vi "test TCX read (installed 71).vi"() -> ()   [LabVIEW 2011] (continued)
sion/v2\"><Watts>118</Watts></TPX></Extensions></Trackpoint><Trackpoint><Time>2008-03-03T13:49:30Z</Time><Position><LatitudeDegrees>35.887382</LatitudeDegrees><LongitudeDegrees>-78.945030</LongitudeDegrees></Position><AltitudeMeters>85.695</AltitudeMeters><DistanceMeters>793.797</DistanceMeters><Cadence>84</Cadence><Extensions><TPX xmlns=\"http://www.garmin.com/xmlschemas/ActivityExtension/v2\"><Watts>105</Watts></TPX></Extensions></Trackpoint><Trackpoint><Time>2008-03-03T13:49:31Z</Time><Position><LatitudeDegrees>35.887368</LatitudeDegrees><LongitudeDegrees>-78.944943</LongitudeDegrees></Position><AltitudeMeters>85.695</AltitudeMeters><DistanceMeters>801.819</DistanceMeters><Cadence>84</Cadence><Extensions><TPX xmlns=\"http://www.garmin.com/xmlschemas/ActivityExtension/v2\"><Watts>104</Watts></TPX></Extensions></Trackpoint><Trackpoint><Time>2008-03-03T13:49:32Z</Time><Position><LatitudeDegrees>35.887352</LatitudeDegrees><LongitudeDegrees>-78.944857</LongitudeDegrees></Position><AltitudeMeters>85.695</AltitudeMeters><DistanceMeters>809.764</DistanceMeters><Cadence>81</Cadence><Extensions><TPX xmlns=\"http://www.garmin.com/xmlschemas/ActivityExtension/v2\"><Watts>123</Watts></TPX></Extensions></Trackpoint><Trackpoint><Time>2008-03-03T13:49:33Z</Time><Position><LatitudeDegrees>35.887335</LatitudeDegrees><LongitudeDegrees>-78.944773</LongitudeDegrees></Position><AltitudeMeters>85.695</AltitudeMeters><DistanceMeters>817.588</DistanceMeters><Cadence>81</Cadence><Extensions><TPX xmlns=\"http://www.garmin.com/xmlschemas/ActivityExtension/v2\"><Watts>122</Watts></TPX></Extensions></Trackpoint><Trackpoint><Time>2008-03-03T13:49:34Z</Time><Position><LatitudeDegrees>35.887319</LatitudeDegrees><LongitudeDegrees>-78.944691</LongitudeDegrees></Position><AltitudeMeters>86.175</AltitudeMeters><DistanceMeters>825.167</DistanceMeters><Cadence>76</Cadence><Extensions><TPX xmlns=\"http://www.garmin.com/xmlschemas/ActivityExtension/v2\"><Watts>160</Watts></TPX></Extensions></Trackpoint><Trackpoint><Time>2008-03-03T13:49:35Z</Time><Position><LatitudeDegrees>35.887303</LatitudeDegrees><LongitudeDegrees>-78.944612</LongitudeDegrees></Position><AltitudeMeters>86.656</AltitudeMeters><DistanceMeters>832.484</DistanceMeters><Cadence>74</Cadence><Extensions><TPX xmlns=\"http://www.garmin.com/xmlschemas/ActivityExtension/v2\"><Watts>198</Watts></TPX></Extensions></Trackpoint><Trackpoint><Time>2008-03-03T13:49:36Z</Time><Position><LatitudeDegrees>35.887288</LatitudeDegrees><LongitudeDegrees>-78.944536</LongitudeDegrees></Position><AltitudeMeters>86.656</AltitudeMeters><DistanceMeters>839.529</DistanceMeters><Cadence>74</Cadence><Extensions><TPX xmlns=\"http://www.garmin.com/xmlschemas/ActivityExtension/v2\"><Watts>196</Watts></TPX></Extensions></Trackpoint><Trackpoint><Time>2008-03-03T13:49:37Z</Time><Position><LatitudeDegrees>35.887275</LatitudeDegrees><LongitudeDegrees>-78.944463</LongitudeDegrees></Position><AltitudeMeters>87.137</AltitudeMeters><DistanceMeters>846.312</DistanceMeters><Cadence>70</Cadence><Extensions><TPX xmlns=\"http://www.garmin.com/xmlschemas/ActivityExtension/v2\"><Watts>222</Watts></TPX></Extensions></Trackpoint><Trackpoint><Time>2008-03-03T13:49:38Z</Time><Position><LatitudeDegrees>35.887261</LatitudeDegrees><LongitudeDegrees>-78.944394</LongitudeDegrees></Position><AltitudeMeters>87.137</AltitudeMeters><DistanceMeters>852.718</DistanceMeters><Cadence>66</Cadence><Extensions><TPX xmlns=\"http://www.garmin.com/xmlschemas/ActivityExtension/v2\"><Watts>181</Watts></TPX></Extensions></Trackpoint><Trackpoint><Time>2008-03-03T13:49:39Z</Time><Position><LatitudeDegrees>35.887248</LatitudeDegrees><LongitudeDegrees>-78.944330</LongitudeDegrees></Position><AltitudeMeters>87.137</AltitudeMeters><DistanceMeters>858.649</DistanceMeters><Cadence>66</Cadence><Extensions><TPX xmlns=\"http://www.garmin.com/xmlschemas/ActivityExtension/v2\"><Watts>181</Watts></TPX></Extensions></Trackpoint><Trackpoint><Time>2008-03-03T13:49:40Z</Time><Position><LatitudeDegrees>35.887233</LatitudeDegrees><LongitudeDegrees>-78.944273</LongitudeDegrees></Position><AltitudeMeters>87.137</AltitudeMeters><DistanceMeters>863.967</DistanceMeters><Cadence>26</Cadence><Extensions><TPX xmlns=\"http://www.garmin.com/xmlschemas/ActivityExtension/v2\"><Watts>4</Watts></TPX></Extensions></Trackpoint><Trackpoint><Time>2008-03-03T13:49:41Z</Time><Position><LatitudeDegrees>35.887206</LatitudeDegrees><LongitudeDegrees>-78.944231</LongitudeDegrees></Position><AltitudeMeters>87.617</AltitudeMeters><DistanceMeters>868.672</DistanceMeters><Cadence>53</Cadence><Extensions><TPX xmlns=\"http://www.garmin.com/xmlschemas/ActivityExtension/v2\"><Watts>162</Watts></TPX></Extensions></Trackpoint><Trackpoint><Time>2008-03-03T13:49:42Z</Time><Position><LatitudeDegrees>35.887168</LatitudeDegrees><LongitudeDegrees>-78.944206</LongitudeDegrees></Position><AltitudeMeters>88.098</AltitudeMeters><DistanceMeters>873.489</DistanceMeters><Cadence>53</Cadence><Extensions><TPX xmlns=\"http://www.garmin.com/xmlschemas/ActivityExtension/v2\"><Watts>215</Watts></TPX></Extensions></Trackpoint><Trackpoint><Time>2008-03-03T13:49:43Z</Time><Position><LatitudeDegrees>35.887123</LatitudeDegrees><LongitudeDegrees>-78.944197</LongitudeDegrees></Position><AltitudeMeters>88.098</AltitudeMeters><DistanceMeters>878.466</DistanceMeters><Cadence>53</Cadence><Extensions><TPX xmlns=\"http://www.garmin.com/xmlschemas/ActivityExtension/v2\"><Watts>227</Watts></TPX></Extensions></Trackpoint><Trackpoint><Time>2008-03-03T13:49:44Z</Time><Position><LatitudeDegrees>35.887076</LatitudeDegrees><LongitudeDegrees>-78.944202</LongitudeDegrees></Position><AltitudeMeters>88.579</AltitudeMeters><DistanceMeters>883.720</DistanceMeters><Cadence>54</Cadence><Extensions><TPX xmlns=\"http://www.garmin.com/xmlschemas/ActivityExtension/v2\"><Watts>313</Watts></TPX></Extensions></Trackpoint><Trackpoint><Time>2008-03-03T13:49:45Z</Time><Position><LatitudeDegrees>35.887028</LatitudeDegrees><LongitudeDegrees>-78.944215</LongitudeDegrees></Position><AltitudeMeters>88.579</AltitudeMeters><DistanceMeters>889.221</DistanceMeters><Cadence>55</Cadence><Extensions><TPX xmlns=\"http://www.garmin.com/xmlschemas/ActivityExtension/v2\"><Watts>319</Watts></TPX></Extensions></Trackpoint><Trackpoint><Time>2008-03-03T13:49:46Z</Time><Position><LatitudeDegrees>35.886978</LatitudeDegrees><LongitudeDegrees>-78.944234</LongitudeDegrees></Position><AltitudeMeters>88.579</AltitudeMeters><DistanceMeters>895.079</DistanceMeters><Cadence>59</Cadence><Extensions><TPX xmlns=\"http://www.garmin.com/xmlschemas/ActivityExtension/v2\"><Watts>307</Watts></TPX></Extensions></Trackpoint><Trackpoint><Time>2008-03-03T13:49:47Z</Time><Position><LatitudeDegrees>35.886925</LatitudeDegrees><LongitudeDegrees>-78.944254</LongitudeDegrees></Position><AltitudeMeters>89.059</AltitudeMeters><DistanceMeters>901.230</DistanceMeters><Cadence>64</Cadence><Extensions><TPX xmlns=\"http://www.garmin.com/xmlschemas/ActivityExtension/v2\"><Watts>315</Watts></TPX></Extensions></Trackpoint><Trackpoint><Time>2008-03-03T13:49:48Z</Time><Position><LatitudeDegrees>35.886870</LatitudeDegrees><LongitudeDegrees>-78.944274</LongitudeDegrees></Position><AltitudeMeters>89.059</AltitudeMeters><DistanceMeters>907.640</DistanceMeters><Cadence>64</Cadence><Extensions><TPX xmlns=\"http://www.garmin.com/xmlschemas/ActivityExtension/v2\"><Watts>314</Watts></TPX></Extensions></Trackpoint><Trackpoint><Time>2008-03-03T13:49:49Z</Time><Position><LatitudeDegrees>35.886813</LatitudeDegrees><LongitudeDegrees>-78.944295</LongitudeDegrees></Position><AltitudeMeters>89.059</AltitudeMeters><DistanceMeters>914.208</DistanceMeters><Cadence>67</Cadence><Extensions><TPX xmlns=\"http://www.garmin.com/xmlschemas/ActivityExtension/v2\"><Watts>312</Watts></TPX></Extensions></Trackpoint><Trackpoint><Time>2008-03-03T13:49:50Z</Time><Position><LatitudeDegrees>35.886755</LatitudeDegrees><LongitudeDegrees>-78.944316</LongitudeDegrees></Position><AltitudeMeters>89.540</AltitudeMeters><DistanceMeters>920.951</DistanceMeters><Cadence>69</Cadence><Extensions><TPX xmlns=\"http://www.garmin.com/xmlschemas/ActivityExtension/v2\"><Watts>307</Watts></TPX></Extensions></Trackpoint><Trackpoint><Time>2008-03-03T13:49:51Z</Time><Position><LatitudeDegrees>35.886696</LatitudeDegrees><LongitudeDegrees>-78.944339</LongitudeDegrees></Position><AltitudeMeters>89.540</AltitudeMeters><DistanceMeters>927.813</DistanceMeters><Cadence>70</Cadence><Extensions><TPX xmlns=\"http://www.garmin.com/xmlschemas/ActivityExtension/v2\"><Watts>284</Watts></TPX></Extensions></Trackpoint><Trackpoint><Time>2008-03-03T13:49:52Z</Time><Position><LatitudeDegrees>35.886636</LatitudeDegrees><LongitudeDegrees>-78.944362</LongitudeDegrees></Position><AltitudeMeters>90.021</AltitudeMeters><DistanceMeters>934.772</DistanceMeters><Cadence>71</Cadence><Extensions><TPX xmlns=\"http://www.garmin.com/xmlschemas/ActivityExtension/v2\"><Watts>269</Watts></TPX></Extensions></Trackpoint><Trackpoint><Time>2008-03-03T13:49:53Z</Time><Position><LatitudeDegrees>35.886575</LatitudeDegrees><LongitudeDegrees>-78.944386</LongitudeDegrees></Position><AltitudeMeters>90.021</AltitudeMeters><DistanceMeters>941.893</DistanceMeters><Cadence>72</Cadence><Extensions><TPX xmlns=\"http://www.garmin.com/xmlschemas/ActivityExtension/v2\"><Watts>267</Watts></TPX></Extensions></Trackpoint><Trackpoint><Time>2008-03-03T13:49:54Z</Time><Position><LatitudeDegrees>35.886513</LatitudeDegrees><LongitudeDegrees>-78.944411</LongitudeDegrees></Position><AltitudeMeters>90.021</AltitudeMeters><DistanceMeters>949.165</DistanceMeters><Cadence>73</Cadence><Extensions><TPX xmlns=\"http://www.garmin.com/xmlschemas/ActivityExtension/v2\"><Watts>268</Watts></TPX></Extensions></Trackpoint><Trackpoint><Time>2008-03-03T13:49:55Z</Time><Position><LatitudeDegrees>35.886450</LatitudeDegrees><LongitudeDegrees>-78.944438</LongitudeDegrees></Position><AltitudeMeters>90.501</AltitudeMeters><DistanceMeters>956.557</DistanceMeters><Cadence>74</Cadence><Extensions><TPX xmlns=\"http://www.garmin.com/xmlschemas/ActivityExtension/v2\"><Watts>281</Watts></TPX></Extensions></Trackpoint><Trackpoint><Time>2008-03-03T13:49:56Z</Time><Position><LatitudeDegrees>35.886386</LatitudeDegrees><LongitudeDegrees>-78.944466</LongitudeDegrees></Position><AltitudeMeters>90.501</AltitudeMeters><DistanceMeters>964.022</DistanceMeters><Cadence>75</Cadence><Extensions><TPX xmlns=\"http://www.garmin.com/xmlschemas/ActivityExtension/v2\"><Watts>280</Watts></TPX></Extensions></Trackpoint><Trackpoint><Time>2008-03-03T13:49:57Z</Time><Position><LatitudeDegrees>35.886323</LatitudeDegrees><LongitudeDegrees>-78.944495</LongitudeDegrees></Position><AltitudeMeters>90.501</AltitudeMeters><DistanceMeters>971.556</DistanceMeters><Cadence>76</Cadence><Extensions><TPX xmlns=\"http://www.garmin.com/xmlschemas/ActivityExtension/v2\"><Watts>255</Watts></TPX></Extensions></Trackpoint><Trackpoint><Time>2008-03-03T13:49:58Z</Time><Position><LatitudeDegrees>35.886260</LatitudeDegrees><LongitudeDegrees>-78.944528</LongitudeDegrees></Position><AltitudeMeters>90.501</AltitudeMeters><DistanceMeters>979.102</DistanceMeters><Cadence>76</Cadence><Extensions><TPX xmlns=\"http://www.garmin.com/xmlschemas/ActivityExtension/v2\"><Watts>221</Watts></TPX></Extensions></Trackpoint><Trackpoint><Time>2008-03-03T13:49:59Z</Time><Position><LatitudeDegrees>35.886198</LatitudeDegrees><LongitudeDegrees>-78.944565</LongitudeDegrees></Position><AltitudeMeters>90.501</AltitudeMeters><DistanceMeters>986.796</DistanceMeters><Cadence>78</Cadence><Extensions><TPX xmlns=\"http://www.garmin.com/xmlschemas/ActivityExtension/v2\"><Watts>223</Watts></TPX></Extensions></Trackpoint><Trackpoint><Time>2008-03-03T13:50:00Z</Time><Position><LatitudeDegrees>35.886135</LatitudeDegrees><LongitudeDegrees>-78.944606</LongitudeDegrees></Position><AltitudeMeters>90.501</AltitudeMeters><DistanceMeters>994.741</DistanceMeters><Cadence>80</Cadence><Extensions><TPX xmlns=\"http://www.garmin.com/xmlschemas/ActivityExtension/v2\"><Watts>218</Watts></TPX></Extensions></Trackpoint><Trackpoint><Time>2008-03-03T13:50:01Z</Time><Position><LatitudeDegrees>35.886071</LatitudeDegrees><LongitudeDegrees>-78.944649</LongitudeDegrees></Position><AltitudeMeters>90.501</AltitudeMeters><DistanceMeters>1002.808</DistanceMeters><Cadence>81</Cadence><Extensions><TPX xmlns=\"http://www.garmin.com/xmlschemas/ActivityExtension/v2\"><Watts>218</Watts></TPX></Extensions></Trackpoint><Trackpoint><Time>2008-03-03T13:50:02Z</Time><Position><LatitudeDegrees>35.886008</LatitudeDegrees><LongitudeDegrees>-78.944696</LongitudeDegrees></Position><AltitudeMeters>90.501</AltitudeMeters><DistanceMeters>1011.004</DistanceMeters><Cadence>77</Cadence><Extensions><TPX xmlns=\"http://www.garmin.com/xmlschemas/ActivityExtension/v2\"><Watts>191</Watts></TPX></Extensions></Trackpoint><Trackpoint><Time>2008-03-03T13:50:03Z</Time><Position><LatitudeDegrees>35.885946</LatitudeDegrees><LongitudeDegrees>-78.944747</LongitudeDegrees></Position><AltitudeMeters>90.501</AltitudeMeters><DistanceMeters>1019.345</DistanceMeters><Cadence>77</Cadence><Extensions><TPX xmlns=\"http://www.garmin.com/xmlschemas/ActivityExtension/v2\"><Watts>191</Watts></TPX></Extensions></Trackpoint><Trackpoint><Time>2008-03-03T13:50:04Z</Time><Position><LatitudeDegrees>35.885883</LatitudeDegrees><LongitudeDegrees>-78.944801</LongitudeDegrees></Position><AltitudeMeters>90.021</AltitudeMeters><DistanceMeters>1027.811</DistanceMeters><Cadence>77</Cadence><Extensions><TPX xmlns=\"http://www.garmin.com/xmlschemas/ActivityExtension/v2\"><Watts>162</Watts></TPX></Extensions></Trackpoint><Trackpoint><Time>2008-03-03T13:50:05Z</Time><Position><LatitudeDegrees>35.885821</LatitudeDegrees><LongitudeDegrees>-78.944859</LongitudeDegrees></Position><AltitudeMeters>90.021</AltitudeMeters><DistanceMeters>1036.483</DistanceMeters><Cadence>77</Cadence><Extensions><TPX xmlns=\"http://www.garmin.com/xmlschemas/ActivityExtension/v2\"><Watts>163</Watts></TPX></Extensions></Trackpoint><Trackpoint><Time>2008-03-03T13:50:06Z</Time><Position><LatitudeDegrees>35.885758</LatitudeDegrees><LongitudeDegrees>-78.944919</LongitudeDegrees></Position><AltitudeMeters>90.021</AltitudeMeters><DistanceMeters>1045.314</DistanceMeters><Cadence>79</Cadence><Extensions><TPX xmlns=\"http://www.garmin.com/xmlschemas/ActivityExtension/v2\"><Watts>162</Watts></TPX></Extensions></Trackpoint><Trackpoint><Time>2008-03-03T13:50:07Z</Time><Position><LatitudeDegrees>35.885695</LatitudeDegrees><LongitudeDegrees>-78.944981</LongitudeDegrees></Position><AltitudeMeters>90.021</AltitudeMeters><DistanceMeters>1054.269</DistanceMeters><Cadence>80</Cadence><Extensions><TPX xmlns=\"http://www.garmin.com/xmlschemas/ActivityExtension/v2\"><Watts>162</Watts></TPX></Extensions></Trackpoint><Trackpoint><Time>2008-03-03T13:50:08Z</Time><Position><LatitudeDegrees>35.885631</LatitudeDegrees><LongitudeDegrees>-78.945045</LongitudeDegrees></Position><AltitudeMeters>90.021</AltitudeMeters><DistanceMeters>1063.442</DistanceMeters><Cadence>82</Cadence><Extensions><TPX xmlns=\"http://www.garmin.com/xmlschemas/ActivityExtension/v2\"><Watts>160</Watts></TPX></Extensions></Trackpoint><Trackpoint><Time>2008-03-03T13:50:09Z</Time><Position><LatitudeDegrees>35.885567</LatitudeDegrees><LongitudeDegrees>-78.945111</LongitudeDegrees></Position><AltitudeMeters>89.540</AltitudeMeters><DistanceMeters>1072.743</DistanceMeters><Cadence>84</Cadence><Extensions><TPX xmlns=\"http://www.garmin.com/xmlschemas/ActivityExtension/v2\"><Watts>146</Watts></TPX></Extensions></Trackpoint><Trackpoint><Time>2008-03-03T13:50:10Z</Time><Position><LatitudeDegrees>35.885502</LatitudeDegrees><LongitudeDegrees>-78.945178</LongitudeDegrees></Position><AltitudeMeters>90.021</AltitudeMeters><DistanceMeters>1082.148</DistanceMeters><Cadence>84</Cadence><Extensions><TPX xmlns=\"http://www.garmin.com/xmlschemas/ActivityExtension/v2\"><Watts>146</Watts></TPX></Extensions></Trackpoint><Trackpoint><Time>2008-03-03T13:50:11Z</Time><Position><LatitudeDegrees>35.885437</LatitudeDegrees><LongitudeDegrees>-78.945246</LongitudeDegrees></Position><AltitudeMeters>89.540</AltitudeMeters><DistanceMeters>1091.624</DistanceMeters><Cadence>85</Cadence><Extensions><TPX xmlns=\"http://www.garmin.com/xmlschemas/ActivityExtension/v2\"><Watts>138</Watts></TPX></Extensions></Trackpoint><Trackpoint><Time>2008-03-03T13:50:12Z</Time><Position><LatitudeDegrees>35.885372</LatitudeDegrees><LongitudeDegrees>-78.945314</LongitudeDegrees></Position><AltitudeMeters>89.059</AltitudeMeters><DistanceMeters>1101.113</DistanceMeters><Cadence>86</Cadence><Extensions><TPX xmlns=\"http://www.garmin.com/xmlschemas/ActivityExtension/v2\"><Watts>124</Watts></TPX></Extensions></Trackpoint><Trackpoint><Time>2008-03-03T13:50:13Z</Time><Position><LatitudeDegrees>35.885306</LatitudeDegrees><LongitudeDegrees>-78.945381</LongitudeDegrees></Position><AltitudeMeters>89.059</AltitudeMeters><DistanceMeters>1110.635</DistanceMeters><Cadence>86</Cadence><Extensions><TPX xmlns=\"http://www.garmin.com/xmlschemas/ActivityExtension/v2\"><Watts>126</Watts></TPX></Extensions></Trackpoint><Trackpoint><Time>2008-03-03T13:50:14Z</Time><Position><LatitudeDegrees>35.885239</LatitudeDegrees><LongitudeDegrees>-78.945447</LongitudeDegrees></Position><AltitudeMeters>88.579</AltitudeMeters><DistanceMeters>1120.112</DistanceMeters><Cadence>86</Cadence><Extensions><TPX xmlns=\"http://www.garmin.com/xmlschemas/ActivityExtension/v2\"><Watts>124</Watts></TPX></Extensions></Trackpoint><Trackpoint><Time>2008-03-03T13:50:15Z</Time><Position><LatitudeDegrees>35.885174</LatitudeDegrees><LongitudeDegrees>-78.945514</LongitudeDegrees></Position><AltitudeMeters>88.579</AltitudeMeters><DistanceMeters>1129.584</DistanceMeters><Cadence>86</Cadence><Extensions><TPX xmlns=\"http://www.garmin.com/xmlschemas/ActivityExtension/v2\"><Watts>124</Watts></TPX></Extensions></Trackpoint><Trackpoint><Time>2008-03-03T13:50:16Z</Time><Position><LatitudeDegrees>35.885109</LatitudeDegrees><LongitudeDegrees>-78.945582</LongitudeDegrees></Position><AltitudeMeters>89.059</AltitudeMeters><DistanceMeters>1139.016</DistanceMeters><Cadence>86</Cadence><Extensions><TPX xmlns=\"http://www.garmin.com/xmlschemas/ActivityExtension/v2\"><Watts>130</Watts></TPX></Extensions></Trackpoint><Trackpoint><Time>2008-03-03T13:50:17Z</Time><Position><LatitudeDegrees>35.885046</LatitudeDegrees><LongitudeDegrees>-78.945649</LongitudeDegrees></Position><AltitudeMeters>90.021</AltitudeMeters><DistanceMeters>1148.277</DistanceMeters><Cadence>85</Cadence><Extensions><TPX xmlns=\"http://www.garmin.com/xmlschemas/ActivityExtension/v2\"><Watts>131</Watts></TPX></Extensions></Trackpoint><Trackpoint><Time>2008-03-03T13:50:18Z</Time><Position><LatitudeDegrees>35.884985</LatitudeDegrees><LongitudeDegrees>-78.945716</LongitudeDegrees></Position><AltitudeMeters>90.982</AltitudeMeters><DistanceMeters>1157.323</DistanceMeters><Cadence>84</Cadence><Extensions><TPX xmlns=\"http://www.garmin.com/xmlschemas/ActivityExtension/v2\"><Watts>135</Watts></TPX></Extensions></Trackpoint><Trackpoint><Time>2008-03-03T13:50:19Z</Time><Position><LatitudeDegrees>35.884925</LatitudeDegrees><LongitudeDegrees>-78.945781</LongitudeDegrees></Position><AltitudeMeters>89.540</AltitudeMeters><DistanceMeters>1166.191</DistanceMeters><Cadence>81</Cadence><Extensions><TPX xmlns=\"http://www.garmin.com/xmlschemas/ActivityExtension/v2\"><Watts>152</Watts></TPX></Extensions></Trackpoint><Trackpoint><Time>2008-03-03T13:50:20Z</Time><Position><LatitudeDegrees>35.884864</LatitudeDegrees><LongitudeDegrees>-78.945844</LongitudeDegrees></Position><AltitudeMeters>90.501</AltitudeMeters><DistanceMeters>1174.987</DistanceMeters><Cadence>81</Cadence><Extensions><TPX xmlns=\"http://www.garmin.com/xmlschemas/ActivityExtension/v2\"><Watts>151</Watts></TPX></Extensions></Trackpoint><Trackpoint><Time>2008-03-03T13:50:21Z</Time><Position><LatitudeDegrees>35.884808</LatitudeDegrees><LongitudeDegrees>-78.945907</LongitudeDegrees></Position><AltitudeMeters>90.021</AltitudeMeters><DistanceMeters>1183.414</DistanceMeters><Cadence>80</Cadence><Extensions><TPX xmlns=\"http://www.garmin.com/xmlschemas/ActivityExtension/v2\"><Watts>178</Watts></TPX></Extensions></Trackpoint><Trackpoint><Time>2008-03-03T13:50:22Z</Time><Position><LatitudeDegrees>35.884755</LatitudeDegrees><LongitudeDegrees>-78.945968</LongitudeDegrees></Position><AltitudeMeters>89.540</AltitudeMeters><DistanceMeters>1191.446</DistanceMeters><Cadence>79</Cadence><Extensions><TPX xmlns=\"http://www.garmin.com/xmlschemas/ActivityExtension/v2\"><Watts>217</Watts></TPX></Extensions></Trackpoint><Trackpoint><Time>2008-03-03T13:50:23Z</Time><Position><LatitudeDegrees>35.884706</LatitudeDegrees><LongitudeDegrees>-78.946030</LongitudeDegrees></Position><AltitudeMeters>90.021</AltitudeMeters><DistanceMeters>1199.238</DistanceMeters><Cadence>78</Cadence><Extensions><TPX xmlns=\"http://www.garmin.com/xmlschemas/ActivityExtension/v2\"><Watts>287</Watts></TPX></Extensions></Trackpoint><Trackpoint><Time>2008-03-03T13:50:24Z</Time><Position><LatitudeDegrees>35.884650</LatitudeDegrees><LongitudeDegrees>-78.946090</LongitudeDegrees></Position><AltitudeMeters>89.540</AltitudeMeters><DistanceMeters>1207.446</DistanceMeters><Cadence>77</Cadence><Extensions><TPX xmlns=\"http://www.garmin.com/xmlschemas/ActivityExtension/v2\"><Watts>289</Watts></TPX></Extensions></Trackpoint><Trackpoint><Time>2008-03-03T13:50:25Z</Time><Position><LatitudeDegrees>35.884592</LatitudeDegrees><LongitudeDegrees>-78.946148</LongitudeDegrees></Position><AltitudeMeters>90.021</AltitudeMeters><DistanceMeters>1215.693</DistanceMeters><Cadence>75</Cadence><Extensions><TPX xmlns=\"http://www.garmin.com/xmlschemas/ActivityExtension/v2\"><Watts>287</Watts></TPX></Extensions></Trackpoint><Trackpoint><Time>2008-03-03T13:50:26Z</Time><Position><LatitudeDegrees>35.884536</LatitudeDegrees><LongitudeDegrees>-78.946205</LongitudeDegrees></Position><AltitudeMeters>90.021</AltitudeMeters><DistanceMeters>1223.751</DistanceMeters><Cadence>73</Cadence><Extensions><TPX xmlns=\"http://www.garmin.com/xmlschemas/ActivityExtension/v2\"><Watts>295</Watts></TPX></Extensions></Trackpoint><Trackpoint><Time>2008-03-03T13:50:27Z</Time><Position><LatitudeDegrees>35.884483</LatitudeDegrees><LongitudeDegrees>-78.946259</LongitudeDegrees></Position><AltitudeMeters>90.021</AltitudeMeters><DistanceMeters>1231.388</DistanceMeters><Cadence>73</Cadence><Extensions><TPX xmlns=\"http://www.garmin.com/xmlschemas/ActivityExtension/v2\"><Watts>296</Watts></TPX></Extensions></Trackpoint><Trackpoint><Time>2008-03-03T13:50:28Z</Time><Position><LatitudeDegrees>35.884431</LatitudeDegrees><LongitudeDegrees>-78.946311</LongitudeDegrees></Position><AltitudeMeters>90.501</AltitudeMeters><DistanceMeters>1238.840</DistanceMeters><Cadence>71</Cadence><Extensions><TPX xmlns=\"http://www.garmin.com/xmlschemas/ActivityExtension/v2\"><Watts>301</Watts></TPX></Extensions></Trackpoint><Trackpoint><Time>2008-03-03T13:50:29Z</Time><Position><LatitudeDegrees>35.884379</LatitudeDegrees><LongitudeDegrees>-78.946362</LongitudeDegrees></Position><AltitudeMeters>90.501</AltitudeMeters><DistanceMeters>1246.250</DistanceMeters><Cadence>69</Cadence><Extensions><TPX xmlns=\"http://www.garmin.com/xmlschemas/ActivityExtension/v2\"><Watts>306</Watts></TPX></Extensions></Trackpoint><Trackpoint><Time>2008-03-03T13:50:30Z</Time><Position><LatitudeDegrees>35.884325</LatitudeDegrees><LongitudeDegrees>-78.946412</LongitudeDegrees></Position><AltitudeMeters>90.501</AltitudeMeters><DistanceMeters>1253.653</DistanceMeters><Cadence>69</Cadence><Extensions><TPX xmlns=\"http://www.garmin.com/xmlschemas/ActivityExtension/v2\"><Watts>304</Watts></TPX></Extensions></Trackpoint><Trackpoint><Time>2008-03-03T13:50:31Z</Time><Position><LatitudeDegrees>35.884272</LatitudeDegrees><LongitudeDegrees>-78.946462</LongitudeDegrees></Position><AltitudeMeters>90.501</AltitudeMeters><DistanceMeters>1261.132</DistanceMeters><Cadence>68</Cadence><Extensions><TPX xmlns=\"http://www.garmin.com/xmlschemas/ActivityExtension/v2\"><Watts>304</Watts></TPX></Extensions></Trackpoint><Trackpoint><Time>2008-03-03T13:50:32Z</Time><Position><LatitudeDegrees>35.884218</LatitudeDegrees><LongitudeDegrees>-78.946508</LongitudeDegrees></Position><AltitudeMeters>90.501</AltitudeMeters><DistanceMeters>1268.362</DistanceMeters><Cadence>68</Cadence><Extensions><TPX xmlns=\"http://www.garmin.com/xmlschemas/ActivityExtension/v2\"><Watts>300</Watts></TPX></Extensions></Trackpoint><Trackpoint><Time>2008-03-03T13:50:33Z</Time><Position><LatitudeDegrees>35.884164</LatitudeDegrees><LongitudeDegrees>-78.946555</LongitudeDegrees></Position><AltitudeMeters>90.982</AltitudeMeters><DistanceMeters>1275.758</DistanceMeters><Cadence>69</Cadence><Extensions><TPX xmlns=\"http://www.garmin.com/xmlschemas/ActivityExtension/v2\"><Watts>268</Watts></TPX></Extensions></Trackpoint><Trackpoint><Time>2008-03-03T13:50:34Z</Time><Position><LatitudeDegrees>35.884108</LatitudeDegrees><LongitudeDegrees>-78.946601</LongitudeDegrees></Position><AltitudeMeters>91.463</AltitudeMeters><DistanceMeters>1283.255</DistanceMeters><Cadence>69</Cadence><Extensions><TPX xmlns=\"http://www.garmin.com/xmlschemas/ActivityExtension/v2\"><Watts>267</Watts></TPX></Extensions></Trackpoint><Trackpoint><Time>2008-03-03T13:50:35Z</Time><Position><LatitudeDegrees>35.884049</LatitudeDegrees><LongitudeDegrees>-78.946643</LongitudeDegrees></Position><AltitudeMeters>91.463</AltitudeMeters><DistanceMeters>1290.863</DistanceMeters><Cadence>70</Cadence><Extensions><TPX xmlns=\"http://www.garmin.com/xmlschemas/ActivityExtension/v2\"><Watts>248</Watts></TPX></Extensions></Trackpoint><Trackpoint><Time>2008-03-03T13:50:36Z</Time><Position><LatitudeDegrees>35.883988</LatitudeDegrees><LongitudeDegrees>-78.946685</LongitudeDegrees></Position><AltitudeMeters>90.982</AltitudeMeters><DistanceMeters>1298.547</DistanceMeters><Cadence>70</Cadence><Extensions><TPX xmlns=\"http://www.garmin.com/xmlschemas/ActivityExtension/v2\"><Watts>211</Watts></TPX></Extensions></Trackpoint><Trackpoint><Time>2008-03-03T13:50:37Z</Time><Position><LatitudeDegrees>35.883926</LatitudeDegrees><LongitudeDegrees>-78.946726</LongitudeDegrees></Position><AltitudeMeters>90.982</AltitudeMeters><DistanceMeters>1306.398</DistanceMeters><Cadence>71</Cadence><Extensions><TPX xmlns=\"http://www.garmin.com/xmlschemas/ActivityExtension/v2\"><Watts>186</Watts></TPX></Extensions></Trackpoint><Trackpoint><Time>2008-03-03T13:50:38Z</Time><Position><LatitudeDegrees>35.883861</LatitudeDegrees><LongitudeDegrees>-78.946762</LongitudeDegrees></Position><AltitudeMeters>91.463</AltitudeMeters><DistanceMeters>1314.315</DistanceMeters><Cadence>72</Cadence><Extensions><TPX xmlns=\"http://www.garmin.com/xmlschemas/ActivityExtension/v2\"><Watts>180</Watts></TPX></Extensions></Trackpoint><Trackpoint><Time>2008-03-03T13:50:39Z</Time><Position><LatitudeDegrees>35.883795</LatitudeDegrees><LongitudeDegrees>-78.946799</LongitudeDegrees></Position><AltitudeMeters>91.463</AltitudeMeters><DistanceMeters>1322.389</DistanceMeters><Cadence>74</Cadence><Extensions><TPX xmlns=\"http://www.garmin.com/xmlschemas/ActivityExtension/v2\"><Watts>176</Watts></TPX></Extensions></Trackpoint><Trackpoint><Time>2008-03-03T13:50:40Z</Time><Position><LatitudeDegrees>35.883727</LatitudeDegrees><LongitudeDegrees>-78.946836</LongitudeDegrees></Position><AltitudeMeters>90.982</AltitudeMeters><DistanceMeters>1330.637</DistanceMeters><Cadence>74</Cadence><Extensions><TPX xmlns=\"http://www.garmin.com/xmlschemas/ActivityExtension/v2\"><Watts>176</Watts></TPX></Extensions></Trackpoint><Trackpoint><Time>2008-03-03T13:50:41Z</Time><Position><LatitudeDegrees>35.883657</LatitudeDegrees><LongitudeDegrees>-78.946872</LongitudeDegrees></Position><AltitudeMeters>90.982</AltitudeMeters><DistanceMeters>1339.048</DistanceMeters><Cadence>76</Cadence><Extensions><TPX xmlns=\"http://www.garmin.com/xmlschemas/ActivityExtension/v2\"><Watts>163</Watts></TPX></Extensions></Trackpoint><Trackpoint><Time>2008-03-03T13:50:42Z</Time><Position><LatitudeDegrees>35.883587</LatitudeDegrees><LongitudeDegrees>-78.946905</LongitudeDegrees></Position><AltitudeMeters>90.501</AltitudeMeters><DistanceMeters>1347.440</DistanceMeters><Cadence>76</Cadence><Extensions><TPX xmlns=\"http://www.garmin.com/xmlschemas/ActivityExtension/v2\"><Watts>139</Watts></TPX></Extensions></Trackpoint><Trackpoint><Time>2008-03-03T13:50:43Z</Time><Position><LatitudeDegrees>35.883514</LatitudeDegrees><LongitudeDegrees>-78.946937</LongitudeDegrees></Position><AltitudeMeters>90.982</AltitudeMeters><DistanceMeters>1355.917</DistanceMeters><Cadence>77</Cadence><Extensions><TPX xmlns=\"http://www.garmin.com/xmlschemas/ActivityExtension/v2\"><Watts>135</Watts></TPX></Extensions></Trackpoint><Trackpoint><Time>2008-03-03T13:50:44Z</Time><Position><LatitudeDegrees>35.883442</LatitudeDegrees><LongitudeDegrees>-78.946965</LongitudeDegrees></Position><AltitudeMeters>90.501</AltitudeMeters><DistanceMeters>1364.402</DistanceMeters><Cadence>77</Cadence><Extensions><TPX xmlns=\"http://www.garmin.com/xmlschemas/ActivityExtension/v2\"><Watts>144</Watts></TPX></Extensions></Trackpoint><Trackpoint><Time>2008-03-03T13:50:45Z</Time><Position><LatitudeDegrees>35.883368</LatitudeDegrees><LongitudeDegrees>-78.946992</LongitudeDegrees></Position><AltitudeMeters>89.540</AltitudeMeters><DistanceMeters>1372.919</DistanceMeters><Cadence>78</Cadence><Extensions><TPX xmlns=\"http://www.garmin.com/xmlschemas/ActivityExtension/v2\"><Watts>135</Watts></TPX></Extensions></Trackpoint><Trackpoint><Time>2008-03-03T13:50:46Z</Time><Position><LatitudeDegrees>35.883293</LatitudeDegrees><LongitudeDegrees>-78.947017</LongitudeDegrees></Position><AltitudeMeters>89.540</AltitudeMeters><DistanceMeters>1381.521</DistanceMeters><Cadence>79</Cadence><Extensions><TPX xmlns=\"http://www.garmin.com/xmlschemas/ActivityExtension/v2\"><Watts>127</Watts></TPX></Extensions></Trackpoint><Trackpoint><Time>2008-03-03T13:50:47Z</Time><Position><LatitudeDegrees>35.883217</LatitudeDegrees><LongitudeDegrees>-78.947041</LongitudeDegrees></Position><AltitudeMeters>89.059</AltitudeMeters><DistanceMeters>1390.210</DistanceMeters><Cadence>79</Cadence><Extensions><TPX xmlns=\"http://www.garmin.com/xmlschemas/ActivityExtension/v2\"><Watts>125</Watts></TPX></Extensions></Trackpoint><Trackpoint><Time>2008-03-03T13:50:48Z</Time><Position><LatitudeDegrees>35.883141</LatitudeDegrees><LongitudeDegrees>-78.947063</LongitudeDegrees></Position><AltitudeMeters>89.059</AltitudeMeters><DistanceMeters>1398.953</DistanceMeters><Cadence>80</Cadence><Extensions><TPX xmlns=\"http://www.garmin.com/xmlschemas/ActivityExtension/v2\"><Watts>133</Watts></TPX></Extensions></Trackpoint><Trackpoint><Time>2008-03-03T13:50:49Z</Time><Position><LatitudeDegrees>35.883064</LatitudeDegrees><LongitudeDegrees>-78.947086</LongitudeDegrees></Position><AltitudeMeters>89.059</AltitudeMeters><DistanceMeters>1407.755</DistanceMeters><Cadence>71</Cadence><Extensions><TPX xmlns=\"http://www.garmin.com/xmlschemas/ActivityExtension/v2\"><Watts>151</Watts></TPX></Extensions></Trackpoint><Trackpoint><Time>2008-03-03T13:50:50Z</Time><Position><LatitudeDegrees>35.882986</LatitudeDegrees><LongitudeDegrees>-78.947109</LongitudeDegrees></Position><AltitudeMeters>89.059</AltitudeMeters><DistanceMeters>1416.616</DistanceMeters><Cadence>71</Cadence><Extensions><TPX xmlns=\"http://www.garmin.com/xmlschemas/ActivityExtension/v2\"><Watts>150</Watts></TPX></Extensions></Trackpoint><Trackpoint><Time>2008-03-03T13:50:51Z</Time><Position><LatitudeDegrees>35.882907</LatitudeDegrees><LongitudeDegrees>-78.947131</LongitudeDegrees></Position><AltitudeMeters>89.059</AltitudeMeters><DistanceMeters>1425.583</DistanceMeters><Cadence>73</Cadence><Extensions><TPX xmlns=\"http://www.garmin.com/xmlschemas/ActivityExtension/v2\"><Watts>160</Watts></TPX></Extensions></Trackpoint><Trackpoint><Time>2008-03-03T13:50:52Z</Time><Position><LatitudeDegrees>35.882828</LatitudeDegrees><LongitudeDegrees>-78.947154</LongitudeDegrees></Position><AltitudeMeters>89.059</AltitudeMeters><DistanceMeters>1434.622</DistanceMeters><Cadence>73</Cadence><Extensions><TPX xmlns=\"http://www.garmin.com/xmlschemas/ActivityExtension/v2\"><Watts>160</Watts></TPX></Extensions></Trackpoint><Trackpoint><Time>2008-03-03T13:50:53Z</Time><Position><LatitudeDegrees>35.882748</LatitudeDegrees><LongitudeDegrees>-78.947176</LongitudeDegrees></Position><AltitudeMeters>89.059</AltitudeMeters><DistanceMeters>1443.746</DistanceMeters><Cadence>73</Cadence><Extensions><TPX xmlns=\"http://www.garmin.com/xmlschemas/ActivityExtension/v2\"><Watts>152</Watts></TPX></Extensions></Trackpoint><Trackpoint><Time>2008-03-03T13:50:54Z</Time><Position><LatitudeDegrees>35.882669</LatitudeDegrees><LongitudeDegrees>-78.947199</LongitudeDegrees></Position><AltitudeMeters>89.059</AltitudeMeters><DistanceMeters>1452.742</DistanceMeters><Cadence>73</Cadence><Extensions><TPX xmlns=\"http://www.garmin.com/xmlschemas/ActivityExtension/v2\"><Watts>143</Watts></TPX></Extensions></Trackpoint><Trackpoint><Time>2008-03-03T13:50:55Z</Time><Position><LatitudeDegrees>35.882590</LatitudeDegrees><LongitudeDegrees>-78.947221</LongitudeDegrees></Position><AltitudeMeters>88.579</AltitudeMeters><DistanceMeters>1461.758</DistanceMeters><Cadence>73</Cadence><Extensions><TPX xmlns=\"http://www.garmin.com/xmlschemas/ActivityExtension/v2\"><Watts>123</Watts></TPX></Extensions></Trackpoint><Trackpoint><Time>2008-03-03T13:50:56Z</Time><Position><LatitudeDegrees>35.882511</LatitudeDegrees><LongitudeDegrees>-78.947243</LongitudeDegrees></Position><AltitudeMeters>88.579</AltitudeMeters><DistanceMeters>1470.765</DistanceMeters><Cadence>73</Cadence><Extensions><TPX xmlns=\"http://www.garmin.com/xmlschemas/ActivityExtension/v2\"><Watts>122</Watts></TPX></Extensions></Trackpoint><Trackpoint><Time>2008-03-03T13:50:57Z</Time><Position><LatitudeDegrees>35.882431</LatitudeDegrees><LongitudeDegrees>-78.947266</LongitudeDegrees></Position><AltitudeMeters>88.579</AltitudeMeters><DistanceMeters>1479.823</DistanceMeters><Cadence>73</Cadence><Extensions><TPX xmlns=\"http://www.garmin.com/xmlschemas/ActivityExtension/v2\"><Watts>122</Watts></TPX></Extensions></Trackpoint><Trackpoint><Time>2008-03-03T13:50:58Z</Time><Position><LatitudeDegrees>35.882350</LatitudeDegrees><LongitudeDegrees>-78.947288</LongitudeDegrees></Position><AltitudeMeters>88.098</AltitudeMeters><DistanceMeters>1489.076</DistanceMeters><Cadence>74</Cadence><Extensions><TPX xmlns=\"http://www.garmin.com/xmlschemas/ActivityExtension/v2\"><Watts>140</Watts></TPX></Extensions></Trackpoint><Trackpoint><Time>2008-03-03T13:50:59Z</Time><Position><LatitudeDegrees>35.882268</LatitudeDegrees><LongitudeDegrees>-78.947310</LongitudeDegrees></Position><AltitudeMeters>88.098</AltitudeMeters><DistanceMeters>1498.384</DistanceMeters><Cadence>76</Cadence><Extensions><TPX xmlns=\"http://www.garmin.com/xmlschemas/ActivityExtension/v2\"><Watts>164</Watts></TPX></Extensions></Trackpoint><Trackpoint><Time>2008-03-03T13:51:00Z</Time><Position><LatitudeDegrees>35.882185</LatitudeDegrees><LongitudeDegrees>-78.947334</LongitudeDegrees></Position><AltitudeMeters>87.617</AltitudeMeters><DistanceMeters>1507.913</DistanceMeters><Cadence>77</Cadence><Extensions><TPX xmlns=\"http://www.garmin.com/xmlschemas/ActivityExtension/v2\"><Watts>196</Watts></TPX></Extensions></Trackpoint><Trackpoint><Time>2008-03-03T13:51:01Z</Time><Position><LatitudeDegrees>35.882100</LatitudeDegrees><LongitudeDegrees>-78.947357</LongitudeDegrees></Position><AltitudeMeters>87.617</AltitudeMeters><DistanceMeters>1517.453</DistanceMeters><Cadence>78</Cadence><Extensions><TPX xmlns=\"http://www.garmin.com/xmlschemas/ActivityExtension/v2\"><Watts>198</Watts></TPX></Extensions></Trackpoint><Trackpoint><Time>2008-03-03T13:51:02Z</Time><Position><LatitudeDegrees>35.882014</LatitudeDegrees><LongitudeDegrees>-78.947381</LongitudeDegrees></Position><AltitudeMeters>87.617</AltitudeMeters><DistanceMeters>1527.243</DistanceMeters><Cadence>79</Cadence><Extensions><TPX xmlns=\"http://www.garmin.com/xmlschemas/ActivityExtension/v2\"><Watts>212</Watts></TPX></Extensions></Trackpoint><Trackpoint><Time>2008-03-03T13:51:03Z</Time><Position><LatitudeDegrees>35.881927</LatitudeDegrees><LongitudeDegrees>-78.947405</LongitudeDegrees></Position><AltitudeMeters>87.137</AltitudeMeters><DistanceMeters>1537.185</DistanceMeters><Cadence>80</Cadence><Extensions><TPX xmlns=\"http://www.garmin.com/xmlschemas/ActivityExtension/v2\"><Watts>197</Watts></TPX></Extensions></Trackpoint><Trackpoint><Time>2008-03-03T13:51:04Z</Time><Position><LatitudeDegrees>35.881840</LatitudeDegrees><LongitudeDegrees>-78.947429</LongitudeDegrees></Position><AltitudeMeters>87.137</AltitudeMeters><DistanceMeters>1547.042</DistanceMeters><Cadence>81</Cadence><Extensions><TPX xmlns=\"http://www.garmin.com/xmlschemas/ActivityExtension/v2\"><Watts>177</Watts></TPX></Extensions></Trackpoint><Trackpoint><Time>2008-03-03T13:51:05Z</Time><Position><LatitudeDegrees>35.881752</LatitudeDegrees><LongitudeDegrees>-78.947454</LongitudeDegrees></Position><AltitudeMeters>86.175</AltitudeMeters><DistanceMeters>1557.075</DistanceMeters><Cadence>82</Cadence><Extensions><TPX xmlns=\"http://www.garmin.com/xmlschemas/ActivityExtension/v2\"><Watts>161</Watts></TPX></Extensions></Trackpoint><Trackpoint><Time>2008-03-03T13:51:06Z</Time><Position><LatitudeDegrees>35.881664</LatitudeDegrees><LongitudeDegrees>-78.947480</LongitudeDegrees></Position><AltitudeMeters>86.175</AltitudeMeters><DistanceMeters>1567.188</DistanceMeters><Cadence>82</Cadence><Extensions><TPX xmlns=\"http://www.garmin.com/xmlschemas/ActivityExtension/v2\"><Watts>161</Watts></TPX></Extensions></Trackpoint><Trackpoint><Time>2008-03-03T13:51:07Z</Time><Position><LatitudeDegrees>35.881575</LatitudeDegrees><LongitudeDegrees>-78.947506</LongitudeDegrees></Position><AltitudeMeters>86.175</AltitudeMeters><DistanceMeters>1577.321</DistanceMeters><Cadence>82</Cadence><Extensions><TPX xmlns=\"http://www.garmin.com/xmlschemas/ActivityExtension/v2\"><Watts>162</Watts></TPX></Extensions></Trackpoint><Trackpoint><Time>2008-03-03T13:51:08Z</Time><Position><LatitudeDegrees>35.881486</LatitudeDegrees><LongitudeDegrees>-78.947532</LongitudeDegrees></Position><AltitudeMeters>85.695</AltitudeMeters><DistanceMeters>1587.506</DistanceMeters><Cadence>83</Cadence><Extensions><TPX xmlns=\"http://www.garmin.com/xmlschemas/ActivityExtension/v2\"><Watts>143</Watts></TPX></Extensions></Trackpoint><Trackpoint><Time>2008-03-03T13:51:09Z</Time><Position><LatitudeDegrees>35.881397</LatitudeDegrees><LongitudeDegrees>-78.947558</LongitudeDegrees></Position><AltitudeMeters>85.695</AltitudeMeters><DistanceMeters>1597.600</DistanceMeters><Cadence>82</Cadence><Extensions><TPX xmlns=\"http://www.garmin.com/xmlschemas/ActivityExtension/v2\"><Watts>161</Watts></TPX></Extensions></Trackpoint><Trackpoint><Time>2008-03-03T13:51:10Z</Time><Position><LatitudeDegrees>35.881307</LatitudeDegrees><LongitudeDegrees>-78.947584</LongitudeDegrees></Position><AltitudeMeters>85.214</AltitudeMeters><DistanceMeters>1607.849</DistanceMeters><Cadence>84</Cadence><Extensions><TPX xmlns=\"http://www.garmin.com/xmlschemas/ActivityExtension/v2\"><Watts>202</Watts></TPX></Extensions></Trackpoint><Trackpoint><Time>2008-03-03T13:51:11Z</Time><Position><LatitudeDegrees>35.881216</LatitudeDegrees><LongitudeDegrees>-78.947611</LongitudeDegrees></Position><AltitudeMeters>85.214</AltitudeMeters><DistanceMeters>1618.290</DistanceMeters><Cadence>85</Cadence><Extensions><TPX xmlns=\"http://www.garmin.com/xmlschemas/ActivityExtension/v2\"><Watts>253</Watts></TPX></Extensions></Trackpoint><Trackpoint><Time>2008-03-03T13:51:12Z</Time><Position><LatitudeDegrees>35.881122</LatitudeDegrees><LongitudeDegrees>-78.947637</LongitudeDegrees></Position><AltitudeMeters>85.214</AltitudeMeters><DistanceMeters>1628.960</DistanceMeters><Cadence>87</Cadence><Extensions><TPX xmlns=\"http://www.g
